vi "Main.vi"() -> ()   [LabVIEW 2017]
panel:
  in  "address":string="192.168.1.7"
  out "text":string
  in  "PRN path":path
  out "error out":errorcluster
  out "data out":string
  in  "timeout ms (25000)":i32
  in  "bytes to read":i32
  in  "mode (standard)":T1(ring)
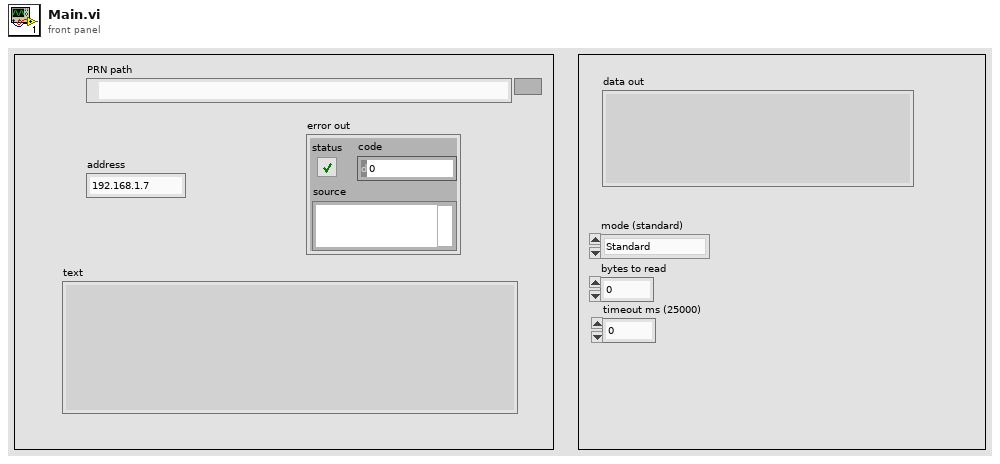
[diagram p1: front panel]
types:
  T1 = enum16{"Standard", "Buffered", "CRLF", "Immediate"}
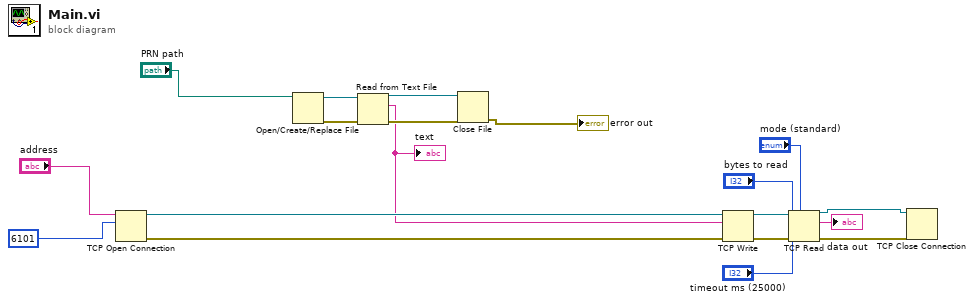
[diagram p0: block diagram]
diagram:
  n1 = TCP Open Connection(address="address", remote port or service name=u16 6101) -> (connection ID=w10:refnum<k5>, error out=w6:errorcluster)  [unwired: 3 in]
  n2 = Open/Create/Replace File(file path (use dialog)="PRN path") -> (refnum out=w7:refnum<file>, error out=w8:errorcluster)  [unwired: 5 in, 1 out]
  n3 = Read from Text File(file (use dialog)=w7, error in=w8) -> (refnum out=w1:refnum<file>, text=w2:string, error out=w4:errorcluster)  [unwired: 2 in, 1 out]
  "text" <- w2
  n4 = Close File(refnum=w1, error in=w4) -> (error out=→"error out":errorcluster)  [unwired: 1 out]
  n5 = TCP Write(connection ID=w10, data in=w2, error in (no error)=w6) -> (connection ID out=w18:refnum<k5>, error out=w19:errorcluster)  [unwired: 1 in, 1 out]
  n6 = TCP Read(connection ID=w18, bytes to read="bytes to read", error in (no error)=w19, 7:"mode (standard)", 9:"timeout ms (25000)") -> (connection ID out=w12:refnum<k5>, data out=→"data out":string, error out=w13:errorcluster)
  n7 = TCP Close Connection(connection ID=w12, error in (no error)=w13) -> ()  [unwired: 1 in, 2 out]
